vi "Auto Global Data.vi"() -> ()   [LabVIEW 2012]
panel:
  in  "Axis Y":dbl
  in  "Axis X":dbl
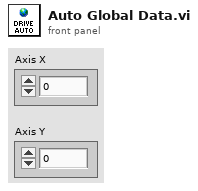
[diagram p1: front panel]
diagram:
